vi "Test program.vi"() -> ()   [LabVIEW 2013, in "Keithly user program.lvlib"]
uses:
  Keithly user program.lvlib
panel:
  out "error out":errorcluster
  out "2182-A Reponse String 2":string
  out "x = y?":bool
  out "Time of one measurement":dbl
  out "2182-A Reponse String":string
  out "2182 -A Params":T1={"Auto Range?"=FALSE, "Man / Selected\n        Range"=0, "Enable Digital\n       Filter?"=FALSE, "Filter Type"=0, "Filter Count"=1, "      Filter\nWindow (%)"=0.01, "Enable Analog\n       Filter?"=FALSE, "NPLCs"=5} {"NPLCs" min=1 max=10; "Filter\nWindow (%)" min=0.01 max=10.0 step=0.01 format="%.2f"; "Filter Count" min=1 max=100; "Filter Type" items=["Movin", "Repeat"]; "Man / Selected\n        Range" items=["10mV", "100mV", "1V", "10V", "100V"]}
  in  "2182 -A Params 3":T2={"Auto Range?"=FALSE, "Man / Selected\n       Range"=enum."10mV", "Enable Digital\n       Filter?"=FALSE, "Filter Type"=enum."Movin", "Filter Count"=1, "      Filter\nWindow (%)"=0.01, "Enable Analog\n       Filter?"=FALSE, "NPLCs"=5} {"NPLCs" min=1 max=10; "Filter\nWindow (%)" min=0.01 max=10.0 step=0.01 format="%.2f"; "Filter Count" min=1 max=100}
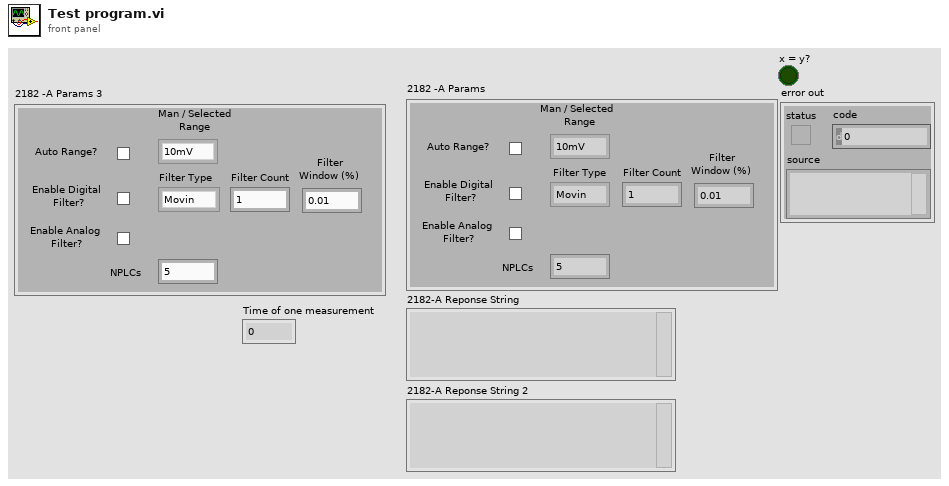
[diagram p1: front panel]
types:
  T1 = cluster{"Auto Range?":bool, "Man / Selected\n        Range":u16, "Enable Digital\n       Filter?":bool, "Filter Type":u16, "Filter Count":u32, "      Filter\nWindow (%)":dbl, "Enable Analog\n       Filter?":bool, "NPLCs":u32}
  T2 = cluster{"Auto Range?":bool, "Man / Selected\n       Range":enum16{"10mV", "100mV", "1V", "10V", "100V"}, "Enable Digital\n       Filter?":bool, "Filter Type":enum16{"Movin", "Repeat"}, "Filter Count":u32, "      Filter\nWindow (%)":dbl, "Enable Analog\n       Filter?":bool, "NPLCs":u32}
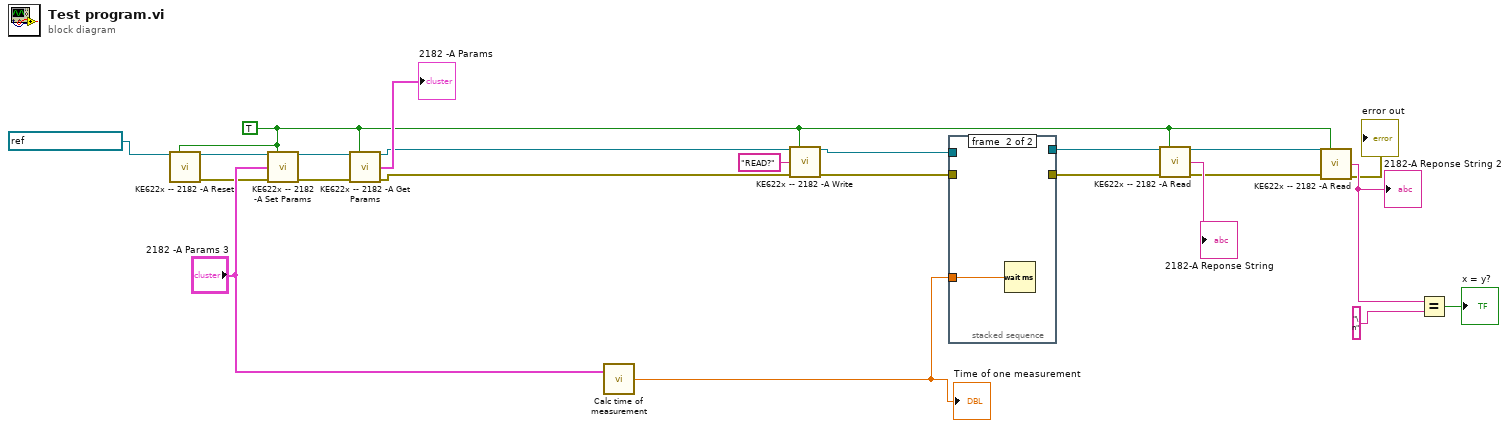
[diagram p0: block diagram]
diagram:
  w2 = TRUE ("Check For SCPI Errors? (T)")
  n1 = call "KE622x -- 2182 -A Reset.vi"("622x Resource In"=refnum<visa-resource-name> "GPIB0::12::INSTR", "Check For SCPI Errors? (T)"=w2) -> ("622x Resource Out (dupl)"=w8:refnum<visa-resource-name>, "error out"=w7:errorcluster)  [unwired: 12 in]
  n2 = call "KE622x -- 2182 -A Set Params.vi"("622x Resource In"=w8, "Check For SCPI Errors? (T)"=w2, "2182 -A Params In"="2182 -A Params 3", "error in (no error)"=w7) -> ("622x Resource Out (dupl)"=w23:refnum<visa-resource-name>, "error out"=w22:errorcluster)  [unwired: 10 in]
  n3 = call "KE622x -- 2182 -A Get Params.vi"("622x Resource In"=w23, "Check For SCPI Errors? (T)"=w2, "error in (no error)"=w22) -> ("622x Resource Out (dupl)"=w18:refnum<visa-resource-name>, "2182 -A Params"=→"2182 -A Params":T1, "error out"=w19:errorcluster)  [unwired: 10 in]
  n4 = call "Calc time of measurement.vi"("2182 -A Params"="2182 -A Params 3") -> ("Time of one measurement"=w11:dbl)  [unwired: 1 in]
  "Time of one measurement" <- w11
  n5 = call "KE622x -- 2182 -A Write.vi"("Resource In"=w18, "Check For SCPI Errors? (T)"=w2, "2182-A Write String"="READ?", "error in (no error)"=w19) -> ("Resource Out (dupl)"=w12:refnum<visa-resource-name>, "error out"=w15:errorcluster)  [unwired: 10 in]
  n6 = stacked-sequence {
    tunnel: w15 -> [w25 _]
    tunnel: [w25 _] -> w14
    tunnel: [w24 _] -> w13
    tunnel: w12 -> [w24 _]
    tunnel: w11 -> [_ w26]
    frame #0 {
    }
    frame #1 {
      n7 = Wait (ms)(milliseconds to wait=w26) -> ()  [unwired: 1 out]
    }
  }
  n8 = call "KE622x -- 2182 -A Read.vi"("622x Resource In"=w13, "Check For SCPI Errors? (T)"=w2, "error in (no error)"=w14) -> ("622x Resource Out (dupl)"=w5:refnum<visa-resource-name>, "2182-A Reponse String"=→"2182-A Reponse String":string, "error out"=w6:errorcluster)  [unwired: 10 in]
  n9 = call "KE622x -- 2182 -A Read.vi"("622x Resource In"=w5, "Check For SCPI Errors? (T)"=w2, "error in (no error)"=w6) -> ("2182-A Reponse String"=w4:string, "error out"=→"error out":errorcluster)  [unwired: 10 in, 1 out]
  "2182-A Reponse String 2" <- w4
  n10 = Equal?(x=w4, y="\n" ("2182-A Reponse String 2")) -> (x = y?=→"x = y?":bool)
